vi "setCamaraSettings.vi"(8 "error in (no error)":errorcluster, 10 "CamaraSettings":refnum<class "CamaraSettings.lvclass">, 11 "Camera in":refnum<class "Camera.lvclass">) -> (0 "error out":errorcluster, 3 "Camera out":refnum<class "Camera.lvclass">)   [LabVIEW 2009, in "Hardware.lvlib" / "Channels.lvlib" / "Camera.lvclass"]
uses:
  Camera.lvclass
  Tools/CameraSettings/CamaraSettings.lvclass
  Camera.lvclass/Camera.ctl
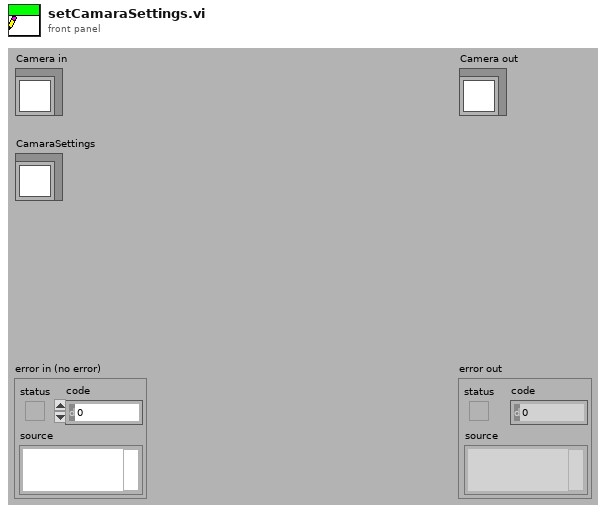
[diagram p1: front panel]
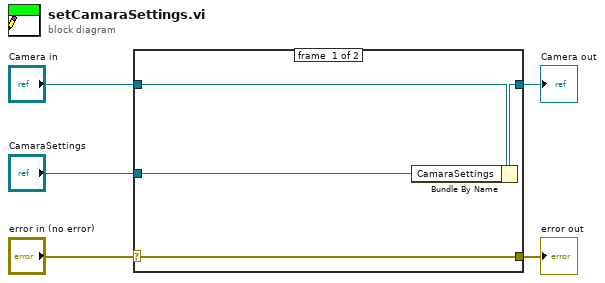
[diagram p0: block diagram]
diagram:
  n1 = case shown="No Error" "error in (no error)" {
    selector: "error in (no error)" -> [w9 w10]
    tunnel: [w9 w10] -> w4
    tunnel: [w7 w11] -> w2
    tunnel: "Camera in" -> [w8 w11]
    tunnel: "CamaraSettings" -> [w6 _]
    frame #0 {
      n2 = Bundle By Name(cluster=w8, "CamaraSettings"=w6) -> (w7:refnum<class "Camera.lvclass">)
    }
    frame #1 {
    }
  }
  "error out" <- w4
  "Camera out" <- w2
